vi "Read Assertion Type.vi"(11 "Banana in":refnum<class "Banana.lvclass">) -> (2 "Assertion Type":T1, 3 "Banana out":refnum<class "Banana.lvclass">)   [LabVIEW 2021]
uses:
  Banana.lvclass/Banana.ctl
  Banana.lvclass
  Assertion Action -- enum.ctl
  Bananas.lvlib
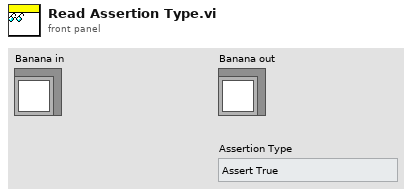
[diagram p1: front panel]
types:
  T1 = typedef "Bananas.lvlib/Assertion Action -- enum.ctl" = enum16{"Assert True", "Assert False"}
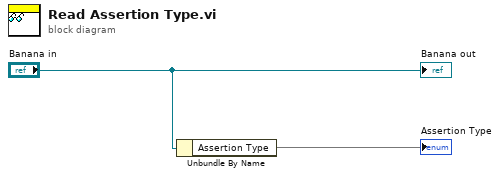
[diagram p0: block diagram]
diagram:
  n1 = Unbundle By Name("Banana in") -> ("Assertion Type"=→"Assertion Type")
  "Banana out" <- "Banana in"
